vi "Update.vi"(8 "error in (no error)":errorcluster, 10 "TimePassed":i64, 11 "UserEventTimer in":refnum<class "TimerEngine.lvclass">) -> (0 "error out":errorcluster, 1 "Cache.TimePeroid(ms)":i32, 2 "Triggered":T1[](array[typedef]), 3 "UserEventTimer out":refnum<class "TimerEngine.lvclass">)   [LabVIEW 2017, in "TimerEngine.lvlib" / "TimerEngine.lvclass"]
uses:
  TimerEngine.lvclass
  _Typedef/Timer-UserEvent.ctl
  TimerEngine.lvclass/TimerEngine.ctl
  _TimerClass/Timer.lvclass
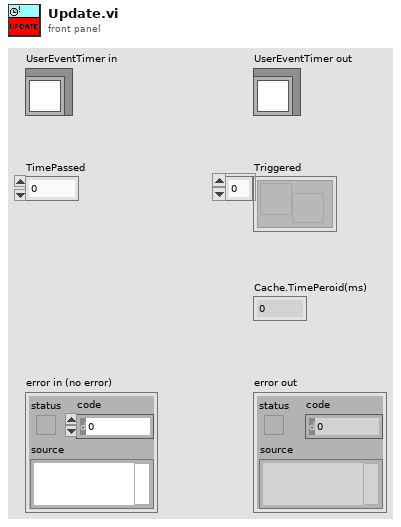
[diagram p1: front panel]
types:
  T1 = typedef "TimerEngine.lvlib/TimerEngine.lvclass/Timer-Userevent.ctl" = refnum<user-event>
  T2 = typedef "TimerEngine.lvlib/TimerEngine.lvclass/Timer-UserEvent.ctl" = refnum<user-event>
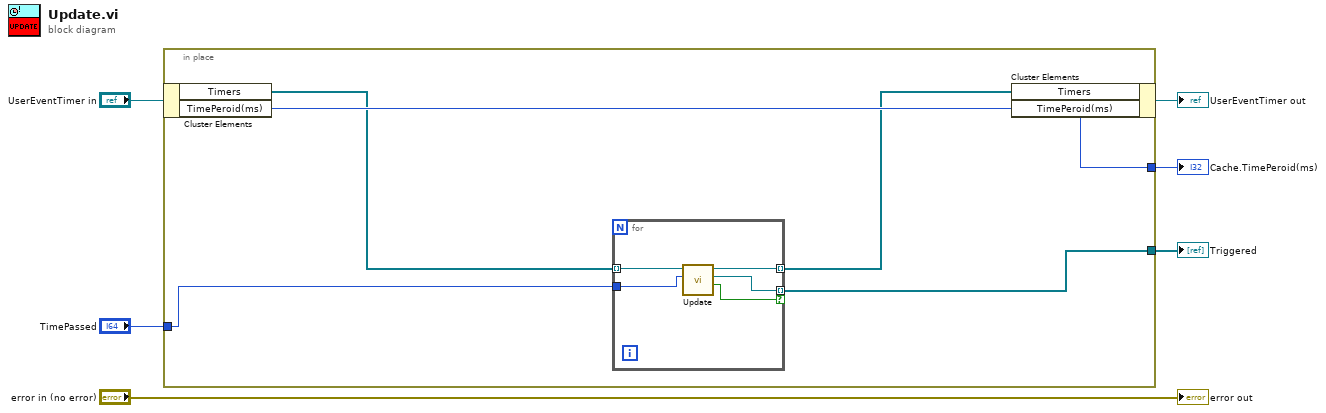
[diagram p0: block diagram]
diagram:
  n1 = in-place "In Place Element Structure" {
    in-place-border: "TimePassed" -> [w8]
    in-place-border: [w11] -> w2
    in-place-border: [w7] -> w1
    n2 = in-place-cluster #1("UserEventTimer in") -> ("Timers"=w10:refnum<class "Timer.lvclass">[], "TimePeroid(ms)"=w11:i64)
    n3 = for {
      tunnel: w10 -> [w16] mode=indexing
      tunnel: [w15] -> w9 mode=indexing
      tunnel: w8 -> [w14]
      tunnel: [w13] -> w7 mode=indexing if=w12
      n4 = call "Update.vi"("TimePassed(ms)"=w14, "Timer in"=w16) -> ("Triggered?"=w12:bool, "UserEvent"=w13:T2, "Timer out"=w15:refnum<class "Timer.lvclass">)  [unwired: 6 in, 1 out]
    }
    n5 = in-place-cluster #1("Timers"=w9, "TimePeroid(ms)"=w11) -> (→"UserEventTimer out":refnum<class "TimerEngine.lvclass">)
  }
  "Triggered" <- w1
  "Cache.TimePeroid(ms)" <- w2
  "error out" <- "error in (no error)"
